vi "Launch as Nested (Parent Task).vi"(8 "error in (no error)":errorcluster, 11 "Parent Task in":refnum<class "Task.lvclass">) -> (0 "error out":errorcluster, 2 "API":refnum<class "DataHandlerAPI.lvclass">, 3 "Parent Task":refnum<class "Task.lvclass">)   [LabVIEW 2020, in "VolatusData.lvlib" / "DataProcessor.lvclass"]
uses:
  DataProcessor.lvclass
  DataHandlerAPI/DataHandlerAPI.lvclass
  C:/dev/lv20CE/relink/lv-volatus/Volatus/API/API.lvclass
  Volatus/Task/Task.lvclass
  C:/dev/lv20CE/relink/lv-volatus/Volatus/Task/Task.lvclass
  C:/dev/lv20CE/relink/lv-volatus/VolatusData/DataHandlerTask/DataHandlerTask.lvclass
  VolatusConfig/VolatusConfigElement/VolatusConfigElement.lvclass/VolatusConfigElement.ctl
  DataProcessor.lvclass/DataProcessor.ctl
  Volatus/Task/Task.lvclass/Task.ctl
  Volatus/VolatusAPI/VolatusAPI.lvclass/VolatusAPI.ctl
  Volatus/Event API/EventAPI.lvclass/EventAPI.ctl
  Volatus/EventHandler Messages/Handle Event Msg/Handle Event Msg.lvclass/Handle Event Msg.ctl
  <vilib>/ActorFramework/Message Enqueuer/Message Enqueuer.lvclass/Message Enqueuer.ctl
  VolatusConfig/VolatusConfigElement/Element.vi
  Volatus/Event API/Report Event.vi
  Volatus/EventHandler Messages/Handle Event Msg/Send Handle Event.vi
  <vilib>/ActorFramework/Message Enqueuer/Enqueue.vi
  VolatusConfig/Task/Task.lvclass
  C:/dev/lv20CE/relink/lv-volatus/VolatusConfig/VolatusConfigElement/VolatusConfigElement.lvclass
  Volatus/EventHandler Messages/Handle Event Msg/Handle Event Msg.lvclass
  C:/Program Files (x86)/National Instruments/LabVIEW 2020/vi.lib/ActorFramework/Message/Message.lvclass
  <vilib>/ActorFramework/Message Priority Queue/Priority Enqueue.vi
  DataHandlerTask/DataHandlerTask.lvclass
  C:/Program Files (x86)/National Instruments/LabVIEW 2020/vi.lib/ActorFramework/Actor/Actor.lvclass
  C:/dev/lv20CE/relink/lv-volatus/Volatus/TaskStateHandler/TaskStateHandler.lvclass
  C:/dev/lv20CE/relink/lv-volatus/Volatus/VectoMessageHandler/VectoMessageHandler.lvclass
  C:/dev/lv20CE/relink/lv-volatus/Volatus/API Provider/API Provider.lvclass
  C:/dev/lv20CE/relink/lv-volatus/VolatusData/DataHandler/DataHandler.lvclass
  C:/dev/lv20CE/relink/lv-volatus/VolatusData/DataProcessor/DataProcessor.lvclass
  C:/dev/lv20CE/relink/lv-volatus/Volatus/Abortable/Abortable.lvclass
  C:/dev/lv20CE/relink/lv-volatus/Volatus/Reconfigurable/Reconfigurable.lvclass
  VolatusConfig/VolatusConfigElement/VolatusConfigElement.lvclass
  C:/dev/lv20CE/relink/lv-volatus/VolatusConfig/Task/Task.lvclass
  C:/dev/lv20CE/relink/lv-volatus/VolatusData/DataHandlerAPI/DataHandlerAPI.lvclass
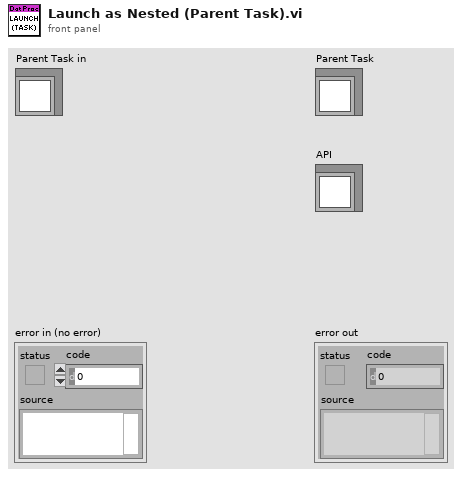
[diagram p1: front panel]
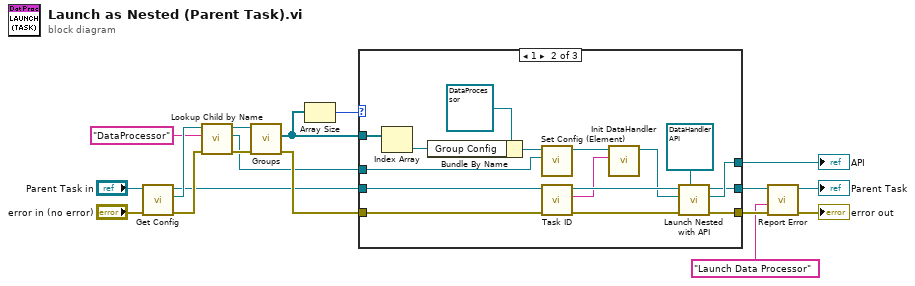
[diagram p0: block diagram]
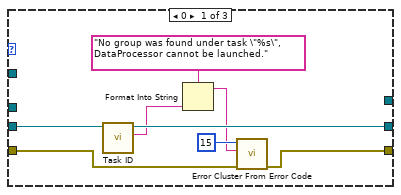
[diagram p2: hidden frame]
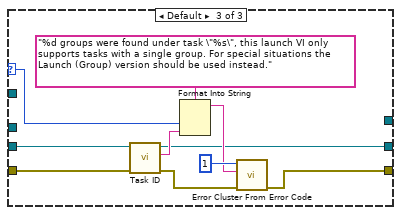
[diagram p3: hidden frame]
diagram:
  n1 = call "Get Config.vi"("error in (no error)"="error in (no error)", "Task in"="Parent Task in") -> ("error out"=w12:errorcluster, "Config"=w10:refnum<class "Task.lvclass">, "Task out"=w4:refnum<class "Task.lvclass">)  [unwired: 7 in]
  n2 = call "Lookup Child by Name.vi"("error in (no error)"=w12, "Child Name"="DataProcessor", "VolatusConfigElement in"=w10) -> ("error out"=w11:errorcluster, "Child"=w3:refnum<class "Config Element.lvclass">, "VolatusConfigElement out"=w9:refnum<class "Task.lvclass">)  [unwired: 5 in, 1 out]
  n3 = call "Groups.vi"("error in (no error)"=w11, "Task in"=w9) -> ("error out"=w5:errorcluster, "Groups"=w2:refnum<class "Group.lvclass">[])  [unwired: 7 in, 1 out]
  n4 = Array Size(array=w2) -> (size(s)=w1:i32)
  n5 = case shown="1" w1 {
    selector: w1 -> [_ _ w51]
    tunnel: [w26 w42 w44] -> w18
    tunnel: [_ w35 _] -> w17
    tunnel: [w22 w32 w43] -> w15
    tunnel: w5 -> [w24 w30 w49]
    tunnel: w4 -> [w23 w29 w50]
    tunnel: w3 -> [_ w28 _]
    tunnel: w2 -> [_ w27 _]
    frame 0 {
      n6 = call-dynamic "Task ID.vi"("Task in"=w23) -> ("Task ID"=w20:string, "Task out"=w22:refnum<class "Task.lvclass">)  [unwired: 8 in, 1 out]
      n7 = Format Into String(format string="No group was found under task \"%s\", DataProcessor cannot be launched.", w20) -> (resulting string=w19:string)  [unwired: 2 in, 1 out]
      n8 = call <vilib>:"Error Cluster From Error Code.vi"("error in (no error)"=w24, "error message (\"\")"=w19, "error code (0)"=15) -> ("error out"=w26:errorcluster)  [unwired: 6 in]
    }
    frame 1 {
      n9 = Index Array(array=w27) -> (element=w31:refnum<class "Group.lvclass">)  [unwired: 1 in]
      n10 = Bundle By Name(cluster=refnum<class "DataProcessor.lvclass"> refnum ("Volatus:DataProcessor.lvclass"), "Group Config"=w31) -> (w33:refnum<class "DataProcessor.lvclass">)
      n11 = call "Set Config (Element).vi"("Config Element"=w28, "Task in"=w33) -> ("Task out"=w34:refnum<class "DataProcessor.lvclass">)  [unwired: 8 in, 1 out]
      n12 = call-dynamic "Task ID.vi"("error in (no error)"=w30, "Task in"=w29) -> ("error out"=w39:errorcluster, "Task ID"=w36:string, "Task out"=w40:refnum<class "Task.lvclass">)  [unwired: 7 in]
      n13 = call "Init DataHandler.vi"("Parent Name"=w36, "DataHandlerTask in"=w34) -> ("DataHandlerTask out"=w37:refnum<class "DataProcessor.lvclass">)  [unwired: 8 in, 1 out]
      n14 = call "Launch Nested with API.vi"("API Type"=refnum<class "DataHandlerAPI.lvclass"> refnum ("Volatus:DataHandlerAPI"), "error in (no error)"=w39, "Nested Task"=w37, "Task in"=w40) -> ("error out"=w42:errorcluster, "API"=w35:refnum<class "DataHandlerAPI.lvclass">, "Task out"=w32:refnum<class "Task.lvclass">)  [unwired: 5 in]
    }
    frame Default {
      n15 = call-dynamic "Task ID.vi"("error in (no error)"=w49, "Task in"=w50) -> ("error out"=w47:errorcluster, "Task ID"=w48:string, "Task out"=w43:refnum<class "Task.lvclass">)  [unwired: 7 in]
      n16 = Format Into String(format string="%d groups were found under task \"%s\", this launch VI only supports tasks with a single group. For special situations the Launch (Group) version should be used instead.", w51, w48) -> (resulting string=w45:string)  [unwired: 2 in, 1 out]
      n17 = call <vilib>:"Error Cluster From Error Code.vi"("error in (no error)"=w47, "error message (\"\")"=w45, "error code (0)"=1) -> ("error out"=w44:errorcluster)  [unwired: 6 in]
    }
  }
  "API" <- w17
  n18 = call "Report Error.vi"("error in (no error)"=w18, "Message"="Launch Data Processor", "Task in"=w15) -> ("error out"=→"error out":errorcluster, "Task out"=→"Parent Task":refnum<class "Task.lvclass">)  [unwired: 7 in]
